vi "transfer open&close door record.vi"(8 "error in (no error)":errorcluster, 11 "isOpenDoor":bool) -> (0 "error out":errorcluster, 3 "response":T1)   [LabVIEW 2016, in "opSignIn.lvlib"]
uses:
  opSignIn.lvlib
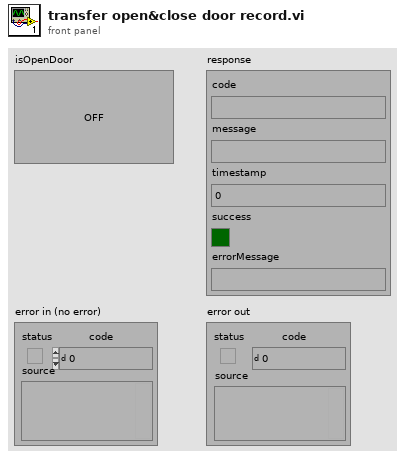
[diagram p1: front panel]
types:
  T1 = cluster{"code":string, "message":string, "timestamp":u64, "success":bool, "errorMessage":string}
  T2 = cluster{"url":string, "AccessToken":string, "mn":string, "isOpenDoor":bool}
  T3 = cluster{"url":string, "loginTokenRequest":cluster{"clientId":string, "clientSecret":string, "grantType":string, "password":string, "scope":string, "userName":string, "userType":string}}
  T4 = cluster{"code":string, "message":string, "timestamp":u64, "data":cluster{"bearerType":string, "oauth2Type":string, "accessToken":string, "tokenType":string, "expiresIn":u64, "refreshToken":string, "scope":string[], "tokenDetail":cluster{"dataSource":string, "username":string, "userId":string, "userType":string, "enabled":bool, "accountNonExpired":bool, "credentialsNonExpired":bool, "accountNonLocked":bool}}, "success":bool}
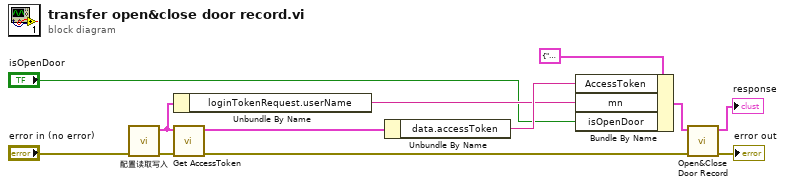
[diagram p0: block diagram]
diagram:
  n1 = call "配置读取写入.vi"("error in (no error)"="error in (no error)") -> ("error out"=w2:errorcluster, "配置输出"=w6:T3)  [unwired: 9 in]
  n2 = Unbundle By Name(w6) -> ("loginTokenRequest.userName"=w10:string)
  n3 = call "Get AccessToken.vi"("error in (no error)"=w2, "配置"=w6) -> ("error out"=w9:errorcluster, "response"=w12:T4)  [unwired: 8 in]
  n4 = Unbundle By Name(w12) -> ("data.accessToken"=w11:string)
  n5 = Bundle By Name(cluster=T2 {"url"="http://dev.watersystem.com.cn:36091", "AccessToken"="equip&4uNDTPGIkWmGoqsxRzBvLK9baeU", "mn"="STDTEST001", "isOpenDoor"=TRUE} ("Para"), "AccessToken"=w11, "mn"=w10, "isOpenDoor"="isOpenDoor") -> (w4:T2)
  n6 = call "Open&Close Door Record.vi"("error in (no error)"=w9, "Para"=w4) -> ("error out"=→"error out":errorcluster, "response"=→"response":T1)  [unwired: 8 in]
